vi "Chroma 1905x Series Configure Hipot High Limit.vi"(4 "Mode":T2 items=["AC", "DC"], 8 "error in (no error)":errorcluster, 9 "Step":T1=1 min=1 max=99 step=1, 10 "Hi Limit [A]":dbl=0.001 min=1e-06 max=0.03 step=1e-06 format="%.3p", 11 "VISA resource name":refnum<visa-resource-name>) -> (0 "error out":errorcluster, 3 "VISA resource name out":refnum<visa-resource-name>)   [LabVIEW 2025]
uses:
  Type Def/modes AC DC--control.ctl
  step--control.ctl
panel:
  # "Configure Hipot High Limit"
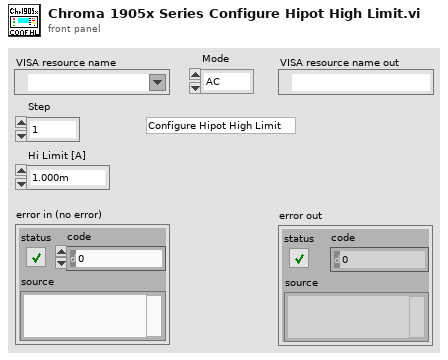
[diagram p1: front panel]
types:
  T1 = typedef "step--control.ctl" = u8
  T2 = typedef "modes AC DC--control.ctl" = i32
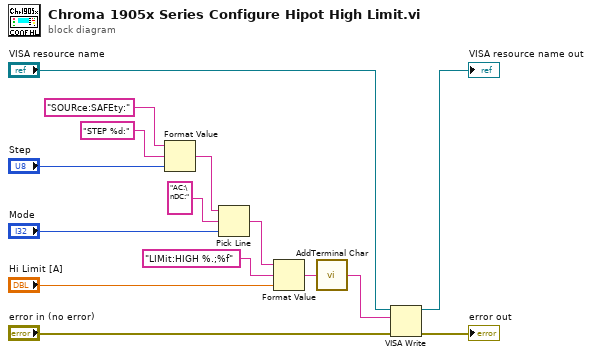
[diagram p0: block diagram]
diagram:
  n1 = Format Value(string ("")="SOURce:SAFEty:", format string="STEP %d:", value (0)="Step") -> (output string=w10:string)
  n2 = Pick Line(string ("")=w10, multi-line string="AC:\nDC:", line index="Mode") -> (output string=w7:string)
  n3 = Format Value(string ("")=w7, format string="LIMit:HIGH %.;%f", value (0)="Hi Limit [A]") -> (output string=w6:string)
  n4 = call "AddTerminal Char.vi"("Cmd string"=w6) -> ("Concatenated String"=w1:string)  [unwired: 4 in]
  n5 = VISA Write(VISA resource name="VISA resource name", write buffer=w1, error in (no error)="error in (no error)") -> (VISA resource name out=→"VISA resource name out":refnum<visa-resource-name>, error out=→"error out":errorcluster)  [unwired: 1 out]
